vi "Tiffs.vi"(2 "Camera Queue":refnum<queue>, 3 "Wave Queue":refnum<queue>) -> (0 "error IO":errorcluster)   [LabVIEW 2016]
uses:
  controls/ModeEnum.ctl
  controls/Microscope Settings.ctl
  controls/CameraControlTypeDef.ctl
  controls/Stack_State.ctl
  controls/Stack Track.ctl
  <vilib>/vision/NI_Vision_Development_Module.lvlib
panel:
  out "FPS":dbl
  out "Numeric":i32
  out "Image":T1(plugin-control)
  in  "Frames":i32
  out "Histogram":T2(graph)
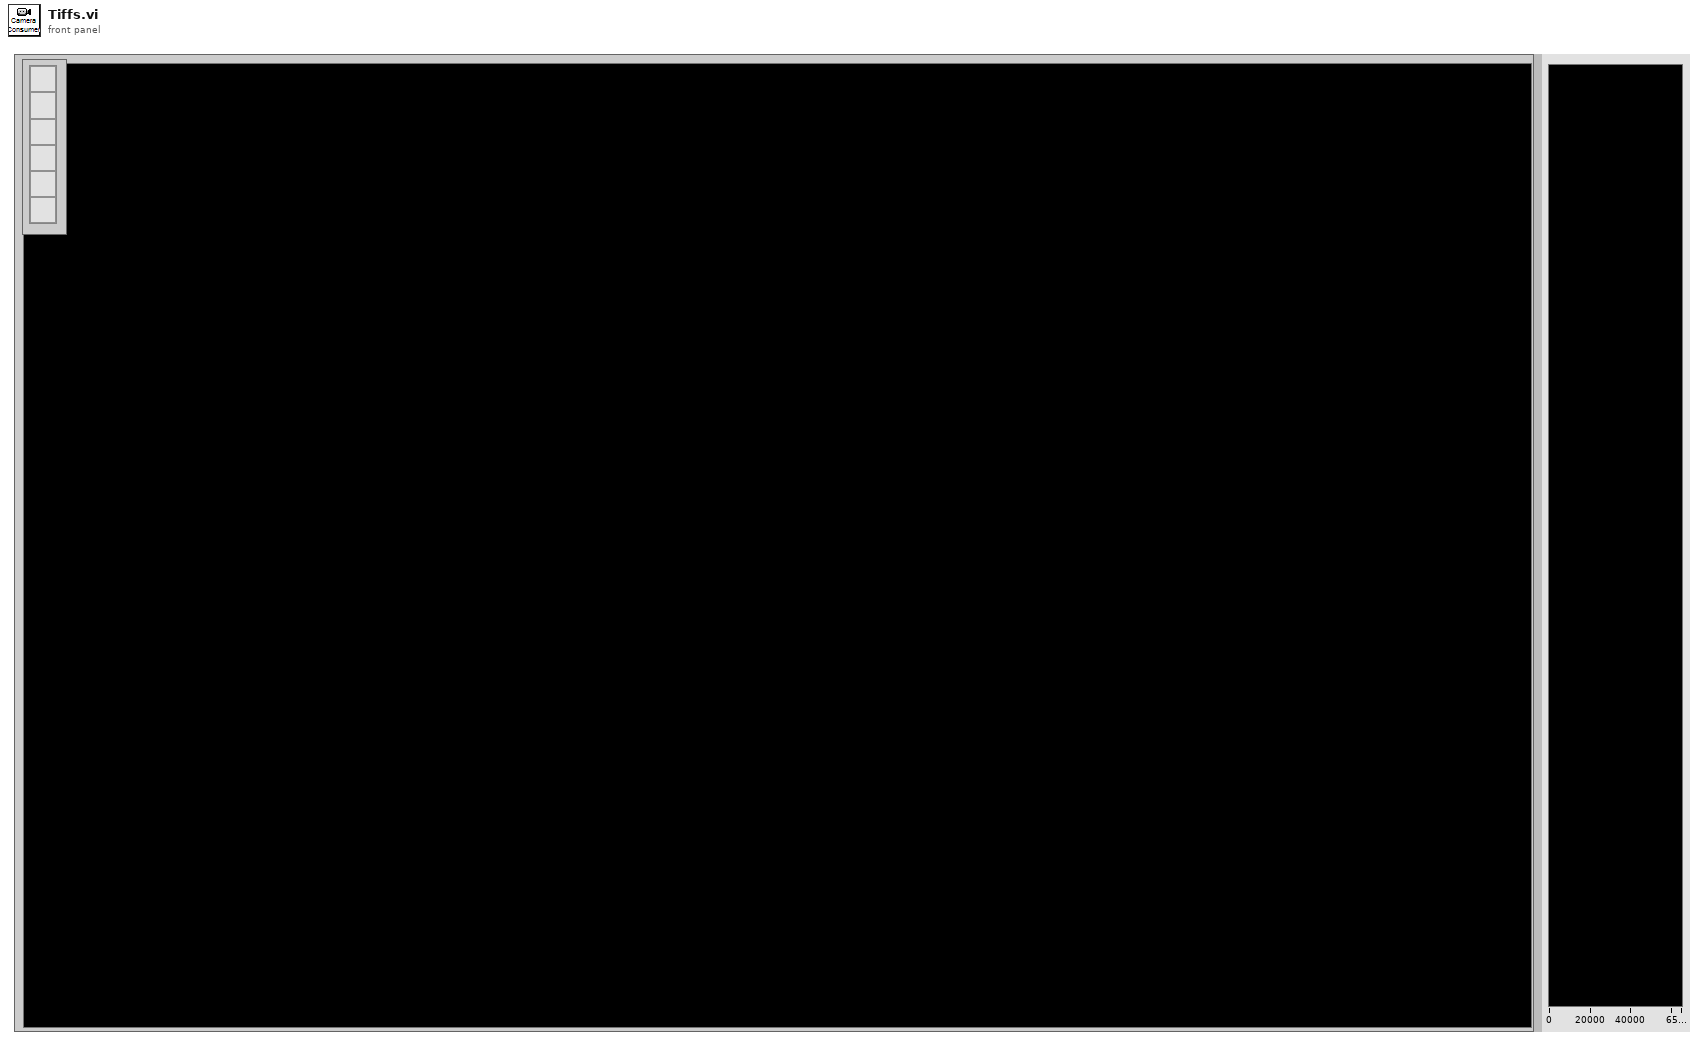
[diagram p1: front panel]
types:
  T1 = typedef "IMAQ Image.ctl" = refnum<image>
  T2 = cluster{"Starting Value":sgl, "Incremental Value":sgl, "Histogram":u32[]}
  T3 = typedef "Stack_State.ctl" = cluster{"State":T4, "Image":u16[][], "Path":path}
  T4 = typedef "Stack Track.ctl" = enum16{"Idle", "STOP", "Display", "Save Image"}
  T5 = typedef "CameraControlTypeDef.ctl" = enum16{"Idle", "Init", "Close", "IntervalLineInt", "Ram Record", "HardDisk Record", "Disengage Update", "Update", "ROI", "Binning", "Scan Mode", "Trigger Mode", "Readout Mode", "Readout Direction", "Preview", "ROIWindow", "Trigger Source"}
  T6 = cluster{"height":u32, "width":u32, "datatype":u32}
  T7 = typedef "Image Type" = u32
  T8 = typedef "Microscope Settings.ctl" = cluster{"Mode":enum16{"Brightfield", "X", "XY", "XYZ", "XYZT", "XYZC", "Tweezers", "Virus"}, "Slit":cluster{"Scanning Mode":dbl, "Slit Width /%":dbl}, "Colour":cluster{"Laser":enum16{"Brightfield", "445", "488", "561", "647"}, "Filter":u16}[], "Exposure/ms":dbl, "Piezo Position /um":dbl, "ROI":cluster{"X":cluster{"Start /px":dbl, "Step /px":dbl, "Range /px":dbl}, "Y":cluster{"Start /px":dbl, "Step /px":dbl, "Range /px":dbl}, "Z ":cluster{"Start /um":dbl, "Step/um":dbl, "Range /um":dbl}, "T ":cluster{"Start /s":dbl, "Step /s":dbl, "Range /s":dbl}}, "Samples per millisecond":dbl, "Relax/ms":dbl, "Readout Direction":dbl, "Trigger Source":dbl, "Camera Delay /ms":dbl, "Under Scan /ms":dbl, "Calibration Coordinates":cluster{"Top Left":dbl[], "Top Right":dbl[], "Bottom Left":dbl[], "Bottom Right":dbl[], "Waveforms":cluster{"Analogue Out":waveform(dbl)[], "Digital Out":digitalwaveform[]}}}
  T9 = typedef "ModeEnum.ctl" = enum16{"Idle", "Init", "generateWaves", "runWaves", "runWavesCont", "endWavesCont", "stop"}
  T10 = cluster{"Mode":u32, "Polarity":u32, "Times":u32, "Delay":dbl}
  T11 = cluster{"State":T4, "Data 16":u16[][], "Save to:":path}
  T12 = enum16{"Brightfield", "X", "XY", "XYZ", "XYZT", "XYZC", "Tweezers", "Virus"}
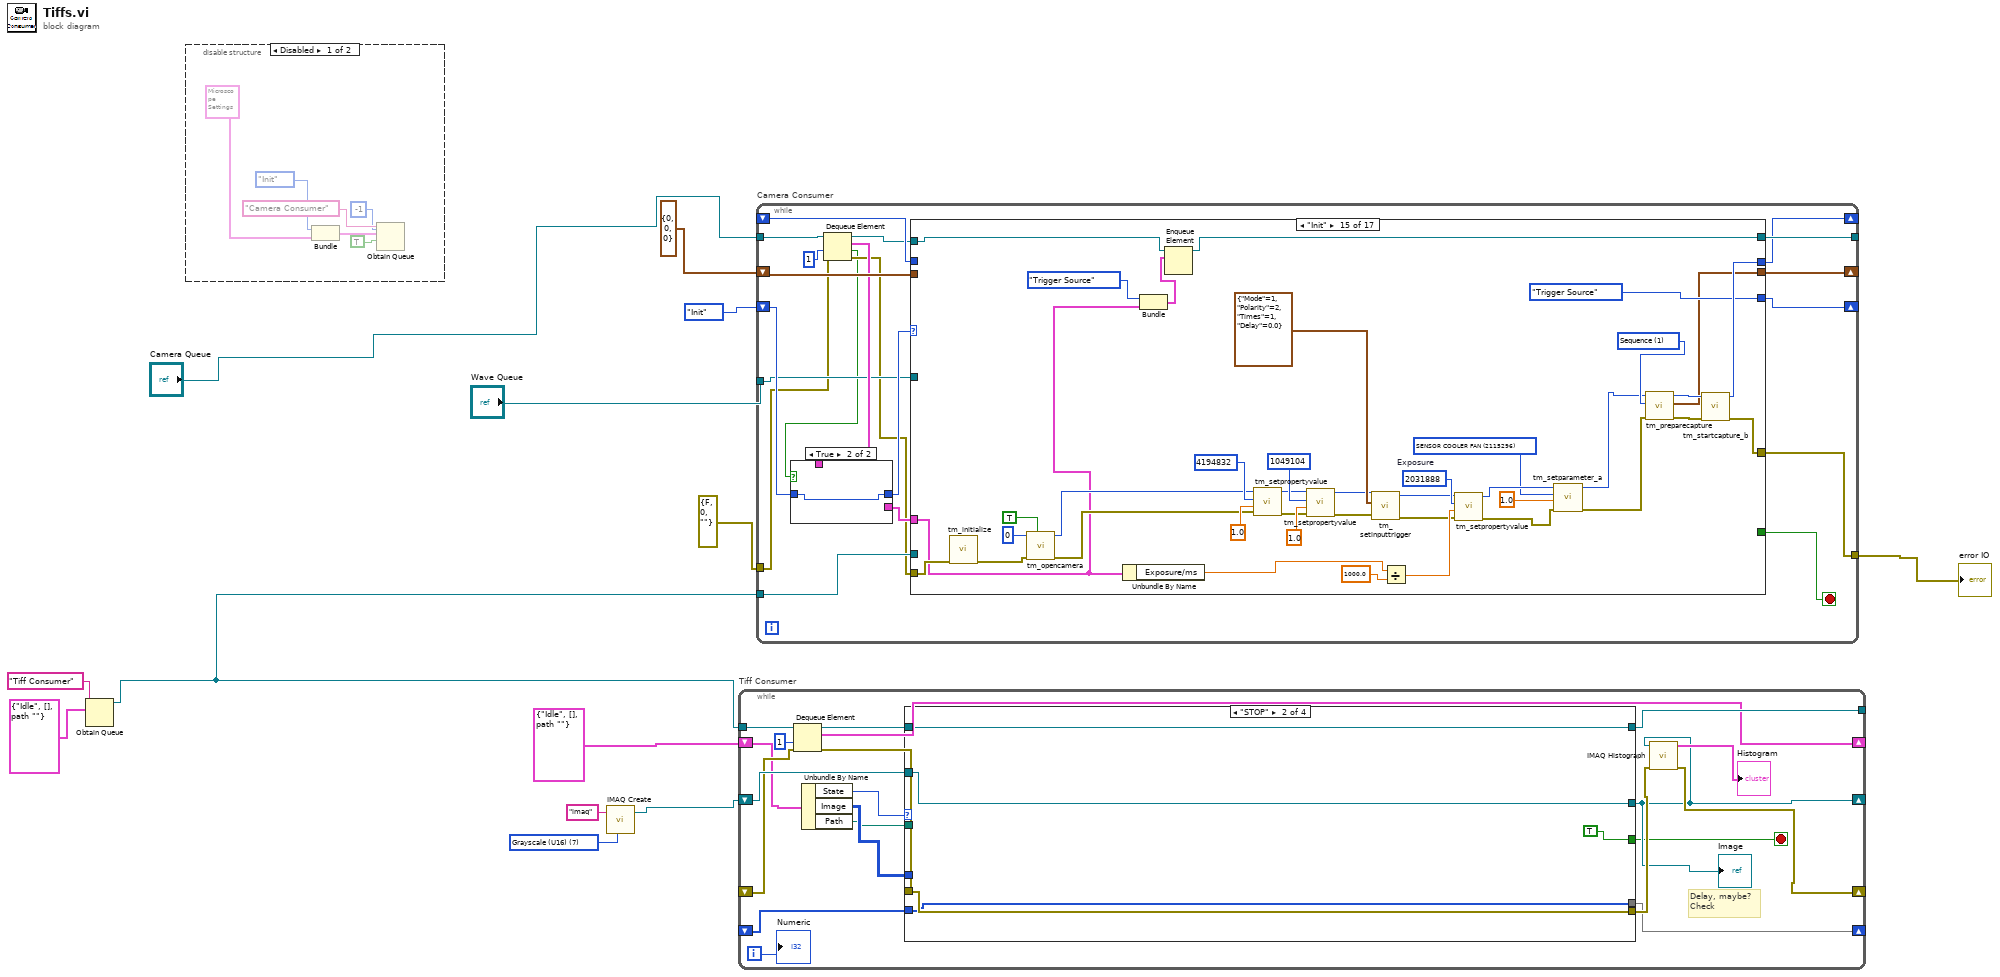
[diagram p0: block diagram]
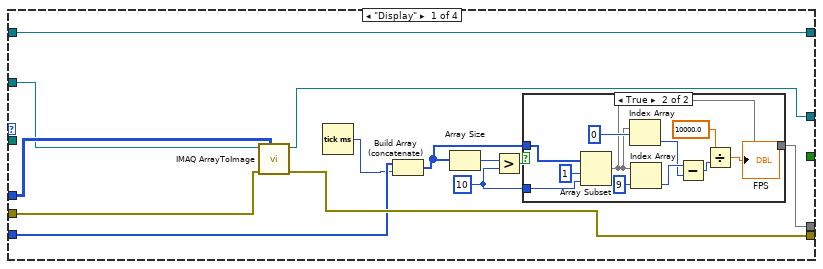
[diagram p3: hidden frame]
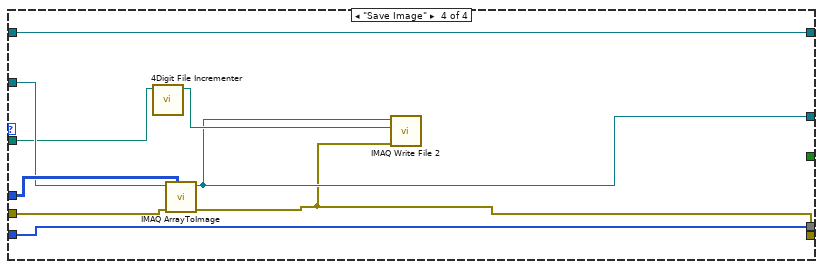
[diagram p6: hidden frame]
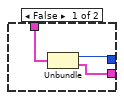
[diagram p7: hidden frame]
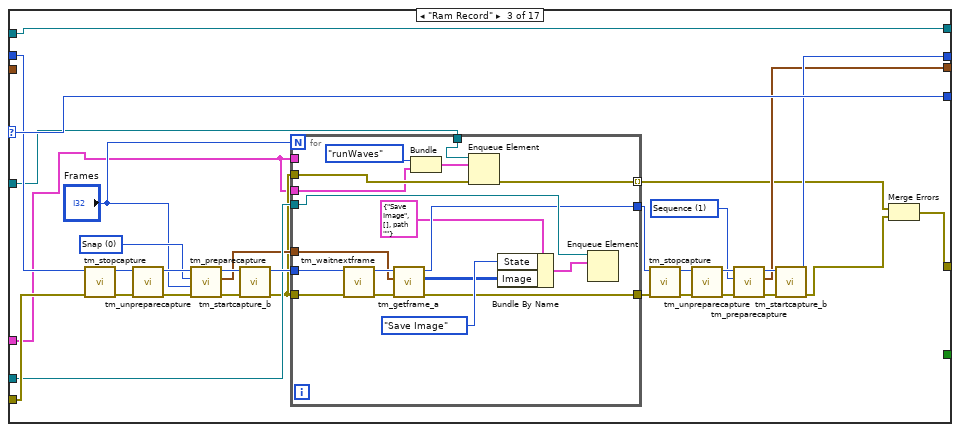
[diagram p10: hidden frame]
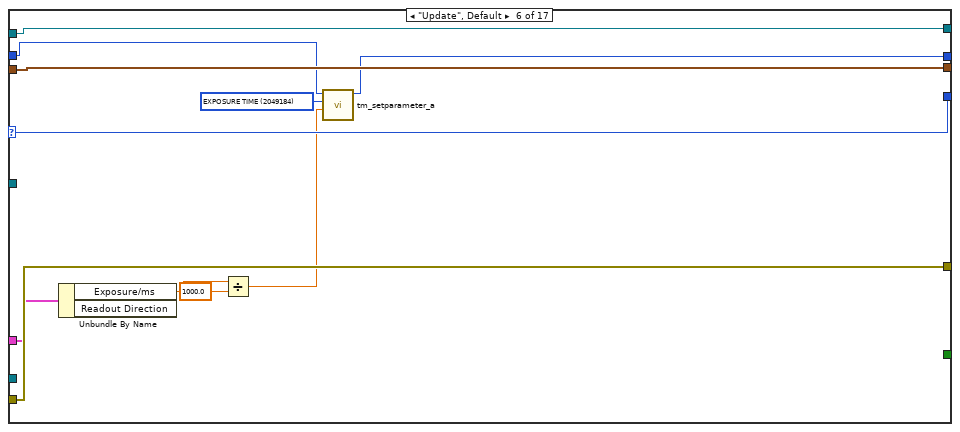
[diagram p13: hidden frame]
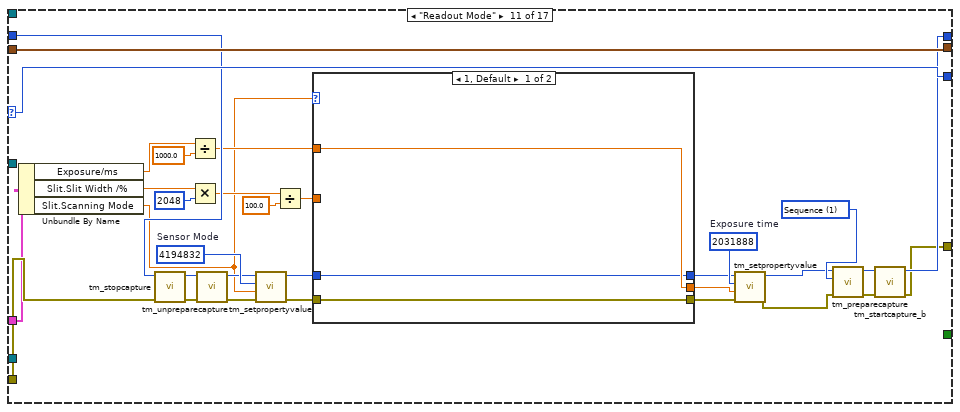
[diagram p18: hidden frame]
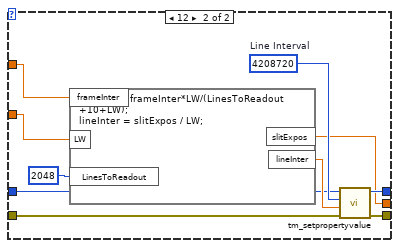
[diagram p19: hidden frame]
diagram:
  w13 = T7 7 items=["Grayscale (U8)", "Grayscale (I16)", "Grayscale (SGL)", "Complex (CSG)", "RGB (U32)", "HSL (U32)", "RGB (U64)", "Grayscale (U16)"] ("Image Type")
  n1 = Obtain Queue(name (unnamed)="Tiff Consumer", element data type=T3 {"State"=enum."Idle", "Image"=[], "Path"=path ""} ("input cluster")) -> (queue out=w1:refnum<queue>)  [unwired: 3 in, 2 out]
  n2 = disable-structure shown="Disabled" {
    frame Disabled {
      n3 = Bundle("Enum"=CameraControlTypeDef."Init", "Microscope Settings"=T8 {"Mode"=enum."X", "Slit"={"Scanning Mode"=12.0, "Slit Width /%"=5.0}, "Colour"=[{"Laser"=enum."561", "Filter"=4}], "Exposure/ms"=40.0, "Piezo Position /um"=0.0, "ROI"={"X"={"Start /px"=0.0, "Step /px"=1.0, "Range /px"=2048.0}, "Y"={"Start /px"=0.0, "Step /px"=1.0, "Range /px"=2048.0}, "Z "={"Start /um"=0.0, "Step/um"=1.0, "Range /um"=100.0}, "T "={"Start /s"=0.0, "Step /s"=1.0, "Range /s"=100.0}}, "Samples per millisecond"=100.0, "Relax/ms"=10.0, "Readout Direction"=2.0, "Trigger Source"=2.0, "Camera Delay /ms"=11.0, "Under Scan /ms"=5.0, "Calibration Coordinates"={"Top Left"=[-4.418670520231216, -0.1592138728323702, 10.0], "Top Right"=[-9.501965317919073, -0.1592138728323702, 10.0], "Bottom Left"=[-4.4508670520231215, 0.0, 0.0], "Bottom Right"=[-9.53757225433526, 0.0, 0.0], "Waveforms"={"Analogue Out"=[], "Digital Out"=[]}}}) -> (w16:cluster{"Enum":T5, "Microscope Settings":T8})  [unwired: 1 in]
      n4 = Obtain Queue(max queue size (-1, unlimited)=-1, name (unnamed)="Camera Consumer", element data type=w16, create if not found? (T)=TRUE) -> ()  [unwired: 1 in, 3 out]
    }
    frame Enabled {
    }
  }
  n5 = call "IMAQ Create"("Image Name"="imaq", "Image Type"=w13) -> ("New Image"=w9:T1)  [unwired: 3 in, 1 out]
  n6 = while "Tiff Consumer" {
    tunnel: [w37] -> _
    tunnel: w1 -> [w38]
    shift-right: [w22] -> _
    shift-left: w9 -> [w31]
    shift-right: [w29] -> _
    shift-left: _ -> [w30]
    shift-right: [w32] -> _
    shift-left: _ -> [w28]
    shift-right: [w26] -> _
    shift-left: T3 {"State"=enum."Idle", "Image"=[], "Path"=path ""} ("input cluster") -> [w25]
    i -> [w27]
    stop <- w20 stop-if-true
    # "Delay, maybe?\nCheck"
    n7 = Dequeue Element(queue=w38, timeout in ms (-1)=1, error in (no error)=w28) -> (queue out=w36:refnum<queue>, element=w26:T3, error out=w35:errorcluster)  [unwired: 1 out]
    n8 = Unbundle By Name(w25) -> ("State"=w34:T4, "Image"=w23:u16[][], "Path"=w21:path)
    n9 = case shown="\"STOP\"" w34 {
      tunnel: [w52 w69 w73 w82] -> w37
      tunnel: w36 -> [w52 w69 w73 w82]
      tunnel: w23 -> [w42 _ _ w81]
      tunnel: w31 -> [w40 w67 w71 w79]
      tunnel: w35 -> [w51 w68 w72 w80]
      tunnel: [w50 w68 w72 w76] -> w33
      tunnel: [w41 w67 w71 w77] -> w22
      tunnel: w30 -> [w49 w66 w70 w75]
      tunnel: [w44 w66 w70 w75] -> w29
      tunnel: w21 -> [_ _ _ w74]
      tunnel: [_ TRUE _ _] -> w20
      frame "Display" {
        w45 = 10 ("y")
        n10 = call "IMAQ ArrayToImage"("Image Pixels (U16)"=w42, "error in (no error)"=w51, "Image"=w40) -> ("error out"=w50:errorcluster, "Image Out"=w41:T1)  [unwired: 7 in]
        n11 = Tick Count (ms)() -> (millisecond timer value=w43:u32)
        n12 = Build Array (concatenate)(w49, w43) -> (w46:u32[])
        n13 = Array Size(array=w46) -> (size(s)=w48:i32)
        n14 = Greater?(x=w48, y=w45) -> (0:w47:bool)
        n15 = case shown="True" w47 {
          tunnel: w46 -> [w53 w56]
          tunnel: w45 -> [_ w63]
          tunnel: [w53 w54] -> w44
          frame False {
          }
          frame True {
            n16 = Array Subset(array=w56, index=1, length=w63) -> (w54:u32[])
            n17 = Index Array(array=w54, index=0) -> (element=w60:u32)
            n18 = Index Array(array=w54, index=9) -> (element=w61:u32)
            n19 = Subtract(x=w61, y=w60) -> (x-y=w59:u32)
            n20 = Divide(x=10000.0, y=w59) -> (x/y=→"FPS":dbl)
          }
        }
      }
      frame "STOP" {
      }
      frame "Idle", Default {
      }
      frame "Save Image" {
        n21 = call "4Digit File Incrementer.vi"("path"=w74) -> ("appended path"=w78:path)  [unwired: 10 in]
        n22 = call "IMAQ ArrayToImage"("Image Pixels (U16)"=w81, "error in (no error)"=w80, "Image"=w79) -> ("error out"=w76:errorcluster, "Image Out"=w77:T1)  [unwired: 7 in]
        n23 = call-poly "IMAQ Write File 2"("error in (no error)"=w76, "File Path"=w78, "Image"=w77) -> ()  [unwired: 7 in, 2 out]
      }
    }
    "Image" <- w22
    n24 = call "IMAQ Histograph"("error in (no error)"=w33, "Image"=w22) -> ("error out"=w32:errorcluster, "Histogram Graph"=→"Histogram":T2)  [unwired: 6 in, 2 out]
    "Numeric" <- w27
  }
  n25 = while "Camera Consumer" {
    tunnel: errorcluster {"status"=FALSE, "code"=0, "source"=""} ("error IO") -> [w85]
    tunnel: [w88] -> w5
    tunnel: "Camera Queue" -> [w95]
    tunnel: [w102] -> _
    shift-right: [w101] -> _
    shift-left: CameraControlTypeDef."Init" ("Enum") -> [w92]
    tunnel: w1 -> [w91]
    shift-right: [w99] -> _
    shift-left: _ -> [w100]
    tunnel: "Wave Queue" -> [w87]
    shift-right: [w98] -> _
    shift-left: T6 {"height"=0, "width"=0, "datatype"=0} ("Buffer Info") -> [w97]
    stop <- w83 stop-if-true
    n26 = Dequeue Element(queue=w95, timeout in ms (-1)=1, error in (no error)=w85) -> (queue out=w94:refnum<queue>, element=w90:cluster{"Enum":T5, "Microscope Settings":T8}, timed out?=w84:bool, error out=w86:errorcluster)
    n27 = case shown="True" w84 {
      tunnel: [w104 w106] -> w93
      tunnel: w92 -> [_ w106]
      tunnel: w90 -> [w105 _]
      tunnel: [w103 _] -> w89
      frame False {
        n28 = Unbundle(w105) -> ("Enum"=w104:T5, "Microscope Settings"=w103:T8)
      }
      frame True {
      }
    }
    n29 = case shown="\"Init\"" w93 {
      selector: w93 -> [w110 w115 w147 w170 w175 w186 w191 w196 w201 w206 w239 w257 _ w286 _ _ _]
      tunnel: w94 -> [w109 w116 w148 w171 w176 w187 w192 w197 w202 w207 _ w253 w268 w288 w292 w338 w366]
      tunnel: [w109 w116 w148 w171 w176 w187 w192 w197 w202 w207 _ w253 w268 w288 w291 _ w366] -> w102
      tunnel: w86 -> [w111 w114 w146 w169 w174 w185 w190 w195 w200 w205 w234 w256 w261 w285 w327 w345 w357]
      tunnel: [w111 w114 w123 w169 w174 w185 w190 w195 w200 w205 w208 w256 w260 w285 w295 w337 w358] -> w88
      tunnel: [w110 w115 w147 w170 w175 w186 w191 w196 w201 w206 w239 w257 CameraControlTypeDef."Preview" ("Enum") w286 CameraControlTypeDef."Trigger Source" ("Enum") CameraControlTypeDef."Idle" ("Enum") w348] -> w101
      tunnel: w100 -> [w108 w113 w130 w168 w172 w183 w189 w194 w199 w204 w236 w255 w267 w287 _ w334 w360]
      tunnel: [w108 w113 w129 w168 w172 w182 w189 w194 w199 w204 w210 w255 w265 w287 w298 w334 w359] -> w99
      tunnel: [w107 w112 w125 w167 w173 w184 w188 w193 w198 w203 w238 w254 w263 w284 w294 w335 w361] -> w98
      tunnel: w97 -> [w107 w112 _ w167 w173 w184 w188 w193 w198 w203 w238 w254 w263 w284 _ w335 _]
      tunnel: w91 -> [_ _ w139 _ _ _ _ _ _ _ _ _ w262 _ _ w328 _]
      tunnel: w89 -> [_ _ w118 _ _ w181 _ _ _ _ w233 _ _ _ w293 _ w350]
      tunnel: w87 -> [_ _ w119 _ _ _ _ _ _ _ _ _ _ _ _ _ _]
      tunnel: [_ _ _ _ _ _ _ _ _ _ _ _ _ _ _ TRUE _] -> w83
      frame "Idle" {
      }
      frame "IntervalLineInt" {
      }
      frame "Ram Record" {
        w143 = 0 items=["Snap", "Sequence"] ("Capture mode")
        w126 = 1 items=["Snap", "Sequence"] ("Capture mode")
        n30 = call <userlib>:"tm_stopcapture.vi"("error in (no error)"=w146, "Handle in"=w130) -> ("error out"=w121:errorcluster, "Handle out"=w122:u32)  [unwired: 8 in]
        n31 = call <userlib>:"tm_unpreparecapture.vi"("error in (no error)"=w121, "Handle in"=w122) -> ("error out"=w145:errorcluster, "Handle out"=w144:u32)  [unwired: 8 in]
        n32 = call <userlib>:"tm_preparecapture.vi"("error in (no error)"=w145, "Frames"="Frames", "Capture mode"=w143, "Handle in"=w144) -> ("error out"=w141:errorcluster, "Buffer Info"=w127:T6, "Handle out"=w142:u32)  [unwired: 4 in, 1 out]
        n33 = call <userlib>:"tm_startcapture_b.vi"("error in (no error)"=w141, "Handle in"=w142) -> ("error out"=w120:errorcluster, "Handle out"=w140:u32)  [unwired: 8 in]
        n34 = for {
          N: "Frames" -> [_]
          tunnel: w120 -> [w166]
          tunnel: w140 -> [w165]
          tunnel: w139 -> [w161]
          tunnel: [w159] -> w135
          tunnel: [w158] -> w134
          tunnel: w127 -> [w157]
          tunnel: w120 -> [w154]
          tunnel: w119 -> [w153]
          tunnel: w118 -> [_]
          tunnel: w118 -> [w151]
          tunnel: [w150] -> w117 mode=indexing
          n35 = call <userlib>:"tm_waitnextframe.vi"("error in (no error)"=w166, "Handle in"=w165) -> ("error out"=w164:errorcluster, "Handle out"=w163:u32)  [unwired: 6 in, 2 out]
          n36 = call <userlib>:"tm_getframe_a.vi"("error in (no error)"=w164, "Buffer Info"=w157, "Handle in"=w163) -> ("error out"=w159:errorcluster, "Data 16"=w155:u16[][], "Handle out"=w158:u32)  [unwired: 4 in, 2 out]
          n37 = Bundle("Mode"=ModeEnum."runWaves", "Microscope Settings"=w151) -> (w149:cluster{"Mode":T9, "Microscope Settings":T8})  [unwired: 1 in]
          n38 = Enqueue Element(queue=w153, element=w149, error in (no error)=w154) -> (error out=w150:errorcluster)  [unwired: 1 in, 2 out]
          n39 = Bundle By Name(cluster=T3 {"State"=enum."Save Image", "Image"=[], "Path"=path ""} ("element"), "State"=Stack_Track."Save Image", "Image"=w155) -> (w160:T3)
          n40 = Enqueue Element(queue=w161, element=w160) -> ()  [unwired: 2 in, 3 out]
        }
        n41 = call <userlib>:"tm_stopcapture.vi"("error in (no error)"=w135, "Handle in"=w134) -> ("error out"=w136:errorcluster, "Handle out"=w133:u32)  [unwired: 8 in]
        n42 = call <userlib>:"tm_unpreparecapture.vi"("error in (no error)"=w136, "Handle in"=w133) -> ("error out"=w137:errorcluster, "Handle out"=w132:u32)  [unwired: 8 in]
        n43 = call <userlib>:"tm_preparecapture.vi"("error in (no error)"=w137, "Capture mode"=w126, "Handle in"=w132) -> ("error out"=w138:errorcluster, "Buffer Info"=w125:T6, "Handle out"=w131:u32)  [unwired: 5 in, 1 out]
        n44 = call <userlib>:"tm_startcapture_b.vi"("error in (no error)"=w138, "Handle in"=w131) -> ("error out"=w124:errorcluster, "Handle out"=w129:u32)  [unwired: 8 in]
        n45 = Merge Errors(w117, w124) -> (w123:errorcluster)
      }
      frame "HardDisk Record" {
      }
      frame "Disengage Update" {
      }
      frame "Update", Default {
        w178 = u32 2049184 items=["SENSOR MODE"=4212128, "CCD MODE"=4212384, "READOUT MODE"=4211872, "ACTIVE VIEW INDEX"=4343136, "BITS PER CHANNEL"=4342976, "IMAGE PIXEL TYPE"=4343296, "BINNING"=4215968, "EXPOSURE TIME"=2049184, "CONTRAST GAIN"=3163312, "CONTRAST OFFSET"=3163328, "LIGHT MODE"=2114720, "SENSITIVITY"=2114992, "PHOTON IMAGING MODE"=2115200, "HIGH DYNAMIC RANGE MODE"=3163360, "WHITE BALANCE"=3163568, "TEMPERATURE"=2115232, "TEMPERATURE TARGET"=2115264, "SENSOR COOLER FAN"=2115296, "LINEBUNDLE HEIGHT"=4212192, "MECHANICAL SHUTTER"=2115488, "BACK FOCUS POSITION"=8422304, "TRIGGER CONNECTOR"=1066432, "TRIGGER SOURCE"=1066144, "OUTPUT TRIGGER SOURCE"=1852576, "TRIGGER GLOBAL EXPOSURE"=2049680, "FIRST TRIGGER BEHAVIOR"=2049696, "CHANNEL SYNC"=1852352, "READOUT DIRECTION"=4211904, "PRE HSYNC COUNT"=1852704, "INTERNAL LINE SPEED"=4226000, "INTERNAL LINE INTERVAL"=4226016] ("Parameter")
        n46 = Unbundle By Name(w181) -> ("Exposure/ms"=w180:dbl)  [unwired: 1 out]
        n47 = Divide(x=w180, y=1000.0) -> (x/y=w177:dbl)
        n48 = call <userlib>:"tm_setparameter_a.vi"("Value in"=w177, "Parameter"=w178, "Handle in"=w183) -> ("Handle out"=w182:u32)  [unwired: 7 in, 1 out]
      }
      frame "ROI" {
      }
      frame "Binning" {
      }
      frame "Scan Mode" {
      }
      frame "Trigger Mode" {
      }
      frame "Readout Mode" {
        w214 = 1 items=["Snap", "Sequence"] ("Capture mode")
        w220 = u32 4194832  # Sensor Mode
        w223 = u32 2031888  # Exposure time
        n49 = Unbundle By Name(w233) -> ("Exposure/ms"=w232:dbl, "Slit.Slit Width /%"=w228:dbl, "Slit.Scanning Mode"=w218:dbl)
        n50 = call <userlib>:"tm_stopcapture.vi"("error in (no error)"=w234, "Handle in"=w236) -> ("error out"=w237:errorcluster, "Handle out"=w235:u32)  [unwired: 8 in]
        n51 = Divide(x=w232, y=1000.0) -> (x/y=w230:dbl)
        n52 = Multiply(x=w228, y=2048 ("input variable")) -> (x*y=w227:dbl)
        n53 = call <userlib>:"tm_unpreparecapture.vi"("error in (no error)"=w237, "Handle in"=w235) -> ("error out"=w215:errorcluster, "Handle out"=w219:u32)  [unwired: 8 in]
        n54 = call "tm_setpropertyvalue.vi"("error in (no error)"=w215, "Value in"=w218, "Property ID"=w220, "Handle in"=w219) -> ("error out"=w216:errorcluster, "Handle out"=w217:u32)  [unwired: 6 in]
        n55 = Divide(x=w227, y=100.0) -> (x/y=w225:dbl)
        n56 = case shown="1, Default" w218 {
          tunnel: [w242 w243] -> w224
          tunnel: w230 -> [w242 w251]
          tunnel: w225 -> [_ w250]
          tunnel: w217 -> [w241 w245]
          tunnel: [w241 w247] -> w222
          tunnel: [w240 w246] -> w221
          tunnel: w216 -> [w240 w244]
          frame 1, Default {
          }
          frame 12 {
            w249 = u32 4208720  # Line Interval
            n57 = formula code="slitExpos=frameInter*LW/(LinesToReadout\n+10+LW);\nlineInter = slitExpos / LW;"("frameInter"=w251, "LW"=w250, "LinesToReadout"=2048 ("input variable")) -> ("slitExpos"=w243:dbl, "lineInter"=w248:dbl)
            n58 = call "tm_setpropertyvalue.vi"("error in (no error)"=w244, "Value in"=w248, "Property ID"=w249, "Handle in"=w245) -> ("error out"=w246:errorcluster, "Handle out"=w247:u32)  [unwired: 6 in]
          }
        }
        n59 = call "tm_setpropertyvalue.vi"("error in (no error)"=w221, "Value in"=w224, "Property ID"=w223, "Handle in"=w222) -> ("error out"=w209:errorcluster, "Handle out"=w211:u32)  [unwired: 6 in]
        n60 = call <userlib>:"tm_preparecapture.vi"("error in (no error)"=w209, "Capture mode"=w214, "Handle in"=w211) -> ("error out"=w213:errorcluster, "Handle out"=w212:u32)  [unwired: 5 in, 2 out]
        n61 = call <userlib>:"tm_startcapture_b.vi"("error in (no error)"=w213, "Handle in"=w212) -> ("error out"=w208:errorcluster, "Handle out"=w210:u32)  [unwired: 8 in]
      }
      frame "Readout Direction" {
      }
      frame "Preview" {
        n62 = call <userlib>:"tm_waitnextframe.vi"("error in (no error)"=w261, "Timeout"=500, "Handle in"=w267) -> ("error out"=w259:errorcluster, "Handle out"=w266:u32)  [unwired: 5 in, 2 out]
        n63 = case shown="No Error" w259 {
          selector: w259 -> [w273 w283]
          tunnel: w266 -> [w281 w282]
          tunnel: [w280 w282] -> w265
          tunnel: w263 -> [w279 _]
          tunnel: w262 -> [w278 _]
          tunnel: w261 -> [w277 _]
          tunnel: [w274 w283] -> w260
          frame No Error {
            n64 = call <userlib>:"tm_getframe_a.vi"("error in (no error)"=w273, "Buffer Info"=w279, "Handle in"=w281) -> ("error out"=w275:errorcluster, "Data 16"=w270:u16[][], "Handle out"=w280:u32)  [unwired: 4 in, 2 out]
            n65 = Bundle("State"=Stack_Track."Display", "Data 16"=w270, "Save to:"=path "C:/_DATA/test.tiff") -> (w269:T11)  [unwired: 1 in]
            n66 = Enqueue Element(queue=w278, element=w269, error in (no error)=w277) -> (error out=w276:errorcluster)  [unwired: 1 in, 2 out]
            n67 = Merge Errors(w275, w276) -> (w274:errorcluster)
          }
          frame Error {
          }
        }
      }
      frame "ROIWindow" {
      }
      frame "Init" {
        w302 = 1 items=["Snap", "Sequence"] ("Capture mode")
        w311 = u32 2115296 items=["SENSOR MODE"=4212128, "CCD MODE"=4212384, "READOUT MODE"=4211872, "ACTIVE VIEW INDEX"=4343136, "BITS PER CHANNEL"=4342976, "IMAGE PIXEL TYPE"=4343296, "BINNING"=4215968, "EXPOSURE TIME"=2049184, "CONTRAST GAIN"=3163312, "CONTRAST OFFSET"=3163328, "LIGHT MODE"=2114720, "SENSITIVITY"=2114992, "PHOTON IMAGING MODE"=2115200, "HIGH DYNAMIC RANGE MODE"=3163360, "WHITE BALANCE"=3163568, "TEMPERATURE"=2115232, "TEMPERATURE TARGET"=2115264, "SENSOR COOLER FAN"=2115296, "LINEBUNDLE HEIGHT"=4212192, "MECHANICAL SHUTTER"=2115488, "BACK FOCUS POSITION"=8422304, "TRIGGER CONNECTOR"=1066432, "TRIGGER SOURCE"=1066144, "OUTPUT TRIGGER SOURCE"=1852576, "TRIGGER GLOBAL EXPOSURE"=2049680, "FIRST TRIGGER BEHAVIOR"=2049696, "CHANNEL SYNC"=1852352, "READOUT DIRECTION"=4211904, "PRE HSYNC COUNT"=1852704, "INTERNAL LINE SPEED"=4226000, "INTERNAL LINE INTERVAL"=4226016] ("Parameter")
        w316 = u32 2031888  # Exposure
        n68 = call <userlib>:"tm_initialize.vi"("error in (no error)"=w327) -> ("error out"=w324:errorcluster)  [unwired: 7 in, 3 out]
        n69 = call <userlib>:"tm_opencamera.vi"("Force Open"=TRUE, "error in (no error)"=w324, "Camera Index"=u32 0) -> ("error out"=w305:errorcluster, "Handle out"=w304:u32)  [unwired: 6 in, 1 out]
        n70 = Unbundle By Name(w293) -> ("Exposure/ms"=w303:dbl)
        n71 = Bundle("Enum"=CameraControlTypeDef."Trigger Source", "Microscope Settings"=w293) -> (w290:cluster{"Enum":T5, "Microscope Settings":T8})  [unwired: 1 in]
        n72 = Enqueue Element(queue=w292, element=w290) -> (queue out=w291:refnum<queue>)  [unwired: 2 in, 2 out]
        n73 = call "tm_setpropertyvalue.vi"("error in (no error)"=w305, "Value in"=sgl 1.0, "Property ID"=u32 4194832, "Handle in"=w304) -> ("error out"=w309:errorcluster, "Handle out"=w319:u32)  [unwired: 6 in]
        n74 = call "tm_setpropertyvalue.vi"("error in (no error)"=w309, "Value in"=sgl 1.0, "Property ID"=u32 1049104, "Handle in"=w319) -> ("error out"=w308:errorcluster, "Handle out"=w317:u32)  [unwired: 6 in]
        n75 = call <userlib>:"tm_setinputtrigger.vi"("error in (no error)"=w308, "Parameters"=T10 {"Mode"=1, "Polarity"=2, "Times"=1, "Delay"=0.0}, "Handle in"=w317) -> ("error out"=w307:errorcluster, "Handle out"=w315:u32)  [unwired: 7 in]
        n76 = Divide(x=w303, y=sgl 1000.0) -> (x/y=w313:dbl)
        n77 = call "tm_setpropertyvalue.vi"("error in (no error)"=w307, "Value in"=w313, "Property ID"=w316, "Handle in"=w315) -> ("error out"=w306:errorcluster, "Handle out"=w312:u32)  [unwired: 6 in]
        n78 = call <userlib>:"tm_setparameter_a.vi"("error in (no error)"=w306, "Value in"=1.0, "Parameter"=w311, "Handle in"=w312) -> ("error out"=w296:errorcluster, "Handle out"=w299:u32)  [unwired: 6 in]
        n79 = call <userlib>:"tm_preparecapture.vi"("error in (no error)"=w296, "Capture mode"=w302, "Handle in"=w299) -> ("error out"=w301:errorcluster, "Buffer Info"=w294:T6, "Handle out"=w300:u32)  [unwired: 5 in, 1 out]
        n80 = call <userlib>:"tm_startcapture_b.vi"("error in (no error)"=w301, "Handle in"=w300) -> ("error out"=w295:errorcluster, "Handle out"=w298:u32)  [unwired: 8 in]
      }
      frame "Close" {
        n81 = Bundle("State"=Stack_Track."STOP", "Data 16"=u16[][] [], "Save to:"=path "C:/_DATA/test.tiff") -> (w330:T11)  [unwired: 1 in]
        n82 = Enqueue Element(queue=w328, element=w330) -> ()  [unwired: 2 in, 3 out]
        n83 = call <userlib>:"tm_stopcapture.vi"("error in (no error)"=w345) -> ("error out"=w344:errorcluster, "Handle out"=w347:u32)  [unwired: 9 in]
        n84 = call <userlib>:"tm_unpreparecapture.vi"("error in (no error)"=w344, "Handle in"=w347) -> ("error out"=w343:errorcluster, "Handle out"=w346:u32)  [unwired: 8 in]
        n85 = call <userlib>:"tm_closecamera.vi"("error in (no error)"=w343, "Handle in"=w346) -> ("error out"=w342:errorcluster)  [unwired: 9 in]
        n86 = call <userlib>:"tm_deinitialize.vi"("error in (no error)"=w342) -> ("error out"=w341:errorcluster)  [unwired: 10 in]
        n87 = Flush Queue(queue=w338, error in (no error)=w341) -> (queue out=w339:refnum<queue>, error out=w340:errorcluster)  [unwired: 1 out]
        n88 = Release Queue(queue=w339, error in (no error)=w340) -> (error out=w337:errorcluster)  [unwired: 1 in, 2 out]
      }
      frame "Trigger Source" {
        (unwired) u32 1066144 items=["SENSOR MODE"=4212128, "CCD MODE"=4212384, "READOUT MODE"=4211872, "ACTIVE VIEW INDEX"=4343136, "BITS PER CHANNEL"=4342976, "IMAGE PIXEL TYPE"=4343296, "BINNING"=4215968, "EXPOSURE TIME"=2049184, "CONTRAST GAIN"=3163312, "CONTRAST OFFSET"=3163328, "LIGHT MODE"=2114720, "SENSITIVITY"=2114992, "PHOTON IMAGING MODE"=2115200, "HIGH DYNAMIC RANGE MODE"=3163360, "WHITE BALANCE"=3163568, "TEMPERATURE"=2115232, "TEMPERATURE TARGET"=2115264, "SENSOR COOLER FAN"=2115296, "LINEBUNDLE HEIGHT"=4212192, "MECHANICAL SHUTTER"=2115488, "BACK FOCUS POSITION"=8422304, "TRIGGER CONNECTOR"=1066432, "TRIGGER SOURCE"=1066144, "OUTPUT TRIGGER SOURCE"=1852576, "TRIGGER GLOBAL EXPOSURE"=2049680, "FIRST TRIGGER BEHAVIOR"=2049696, "CHANNEL SYNC"=1852352, "READOUT DIRECTION"=4211904, "PRE HSYNC COUNT"=1852704, "INTERNAL LINE SPEED"=4226000, "INTERNAL LINE INTERVAL"=4226016] ("Parameter")
        w356 = 1 items=["Snap", "Sequence"] ("Capture mode")
        n89 = Unbundle By Name(w350) -> ("Mode"=w349:T12)
        n90 = call <userlib>:"tm_stopcapture.vi"("error in (no error)"=w357, "Handle in"=w360) -> ("error out"=w364:errorcluster, "Handle out"=w365:u32)  [unwired: 8 in]
        n91 = call <userlib>:"tm_unpreparecapture.vi"("error in (no error)"=w364, "Handle in"=w365) -> ("error out"=w352:errorcluster, "Handle out"=w355:u32)  [unwired: 8 in]
        n92 = case shown="\"Brightfield\"" w349 {
          tunnel: [T10 {"Mode"=2, "Polarity"=2, "Times"=2, "Delay"=0.0} ("Parameters") T10 {"Mode"=2, "Polarity"=2, "Times"=2, "Delay"=0.0} ("Parameters") T10 {"Mode"=2, "Polarity"=2, "Times"=2, "Delay"=0.0} ("Parameters") T10 {"Mode"=1, "Polarity"=2, "Times"=2, "Delay"=0.0} ("Parameters") T10 {"Mode"=1, "Polarity"=2, "Times"=2, "Delay"=0.0} ("Parameters") T10 {"Mode"=1, "Polarity"=2, "Times"=2, "Delay"=0.0} ("Parameters")] -> w353
          tunnel: [CameraControlTypeDef."Preview" ("Enum") CameraControlTypeDef."Idle" ("Enum") CameraControlTypeDef."Idle" ("Enum") CameraControlTypeDef."Idle" ("Enum") CameraControlTypeDef."Preview" ("Enum") CameraControlTypeDef."Preview" ("Enum")] -> w348
          frame "XY", Default {
          }
          frame "XYZT" {
          }
          frame "XYZ" {
          }
          frame "XYZC" {
          }
          frame "X" {
          }
          frame "Brightfield" {
          }
        }
        n93 = call <userlib>:"tm_setinputtrigger.vi"("error in (no error)"=w352, "Parameters"=w353, "Handle in"=w355) -> ("error out"=w351:errorcluster, "Handle out"=w354:u32)  [unwired: 7 in]
        n94 = call <userlib>:"tm_preparecapture.vi"("error in (no error)"=w351, "Capture mode"=w356, "Handle in"=w354) -> ("error out"=w363:errorcluster, "Buffer Info"=w361:T6, "Handle out"=w362:u32)  [unwired: 5 in, 1 out]
        n95 = call <userlib>:"tm_startcapture_b.vi"("error in (no error)"=w363, "Handle in"=w362) -> ("error out"=w358:errorcluster, "Handle out"=w359:u32)  [unwired: 8 in]
      }
    }
  }
  "error IO" <- w5
